vi "esp_kártya_olvasó.vi"() -> ()   [LabVIEW 2015]
uses:
  <vilib>/httpClient/POSTBuffer.vi
  <vilib>/httpClient/LabVIEWHTTPClient.lvlib
panel:
  in  "Tab Control":T1(tab)
  out "value":T2(array[cluster])
  in  "Felhasználó létrehozása":bool
  in  "Felhasználó mentése":T3
  in  "Felhasználó módosítása":bool
  in  "Felhasználó hozzáadása":T3
  out "value 2":cluster{"RFID-code":string, "time":string}[](array[cluster])
  out "Array":string[](array[string])
  out "error out":errorcluster
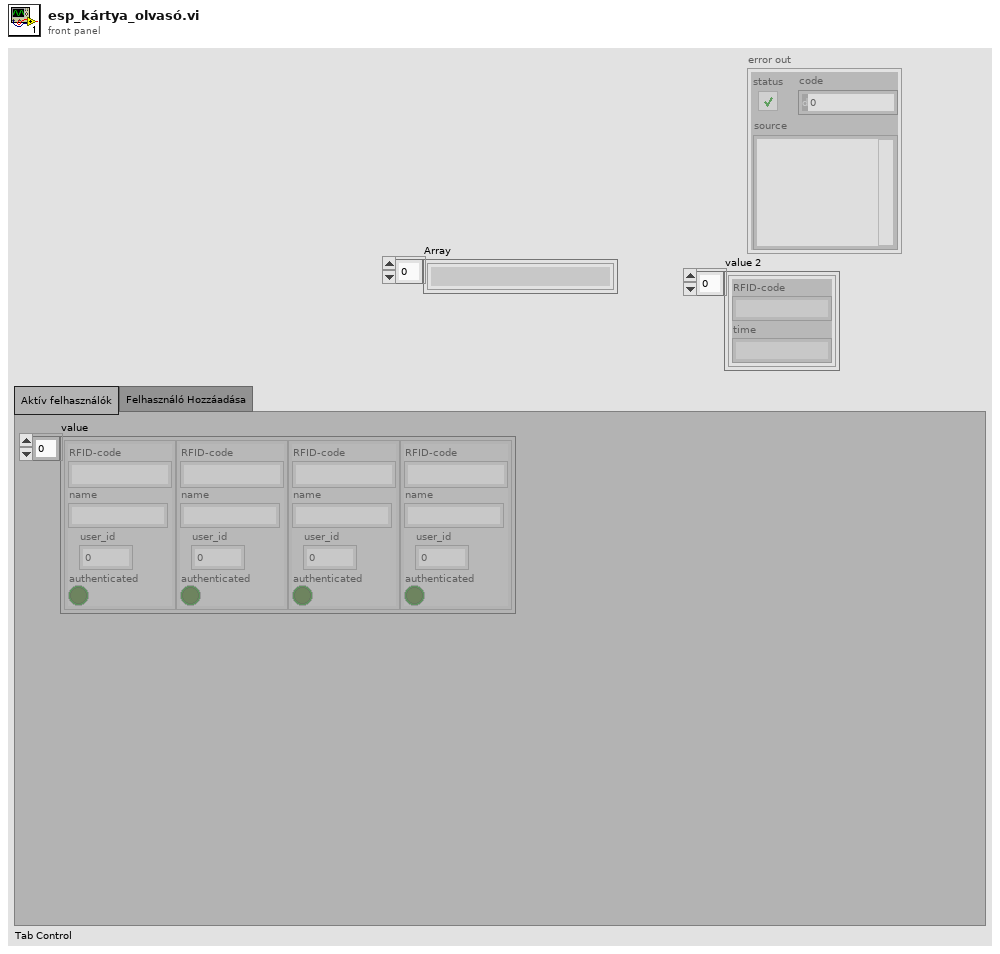
[diagram p1: front panel]
types:
  T1 = enum32{"Aktív felhasználók", "Felhasználó Hozzáadása"}
  T2 = cluster{"RFID-code":string, "name":string, "user_id":dbl, "authenticated":bool}[]
  T3 = cluster{"RFID-code":string, "name":string, "user_id":dbl, "authenticated":bool}
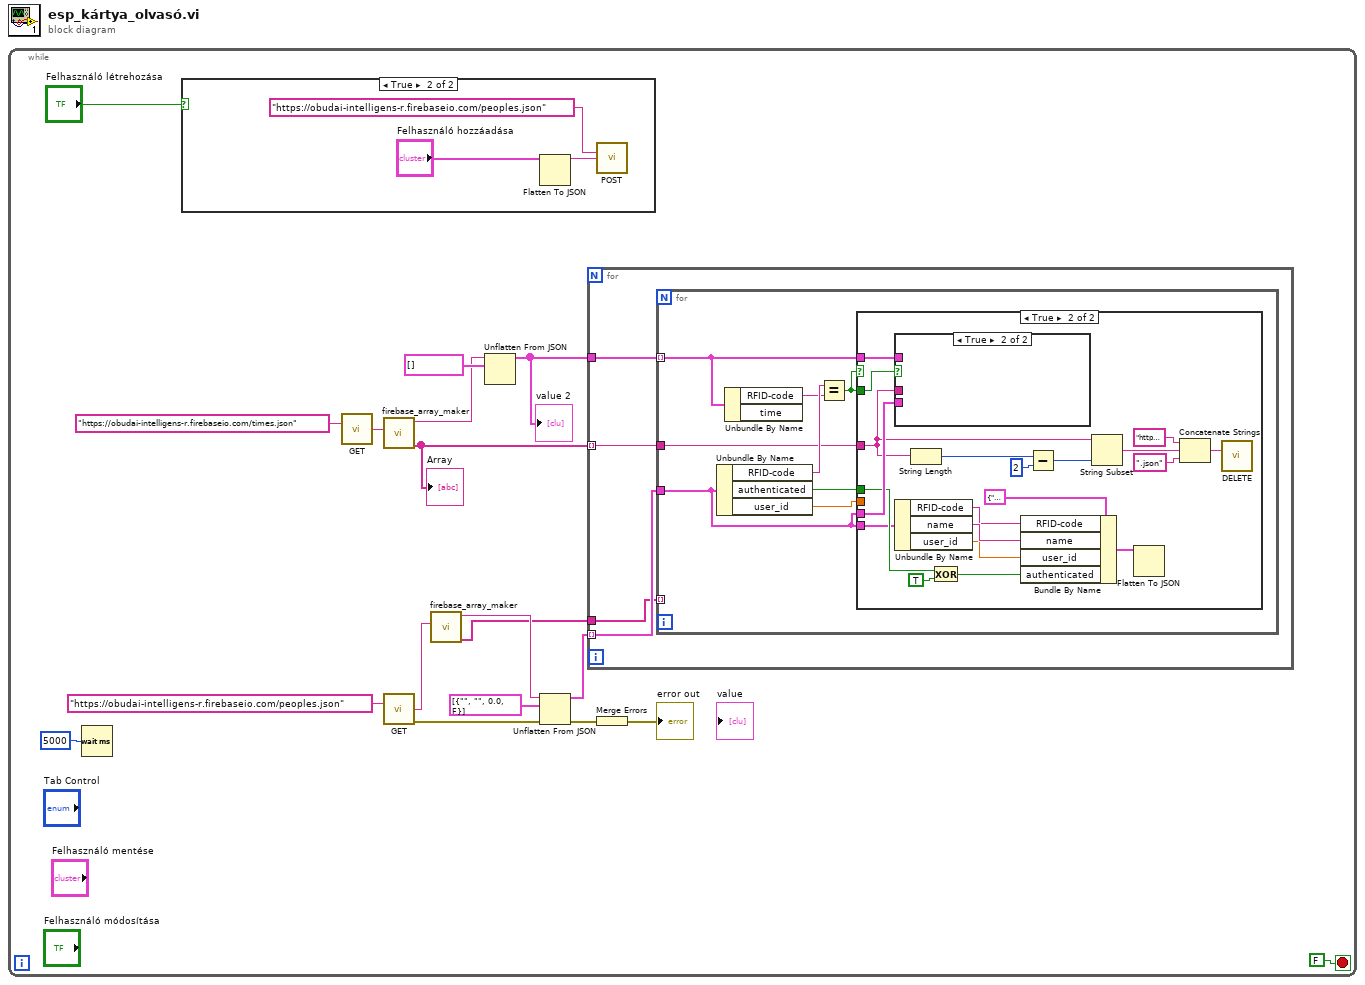
[diagram p0: block diagram]
diagram:
  n1 = while {
    stop <- FALSE stop-if-true
    n2 = Wait (ms)(milliseconds to wait=u32 5000) -> ()  [unwired: 1 out]
    n3 = case shown="True" "Felhasználó létrehozása" {
      frame False {
      }
      frame True {
        n4 = Flatten To JSON(anything="Felhasználó hozzáadása") -> (JSON string=w19:string)  [unwired: 2 in, 1 out]
        n5 = call-poly <vilib>:"POST.vi"("url"="https://obudai-intelligens-r.firebaseio.com/peoples.json", "buffer"=w19) -> ()  [unwired: 10 in, 4 out]
      }
    }
    n6 = call <vilib>:"GET.vi"("url"="https://obudai-intelligens-r.firebaseio.com/times.json") -> ("body"=w6:string)  [unwired: 11 in, 3 out]
    n7 = call "firebase_array_maker.vi"("be_string"=w6) -> ("indexek_ nevei"=w4:string[], "json ki"=w5:string)  [unwired: 9 in]
    "Array" <- w4
    n8 = call <vilib>:"GET.vi"("url"="https://obudai-intelligens-r.firebaseio.com/peoples.json") -> ("body"=w2:string, "error out"=w17:errorcluster)  [unwired: 11 in, 2 out]
    n9 = call "firebase_array_maker.vi"("be_string"=w2) -> ("indexek_ nevei"=w1:string[], "json ki"=w3:string)  [unwired: 9 in]
    n10 = Unflatten From JSON(JSON string=w5, type and defaults=cluster{"RFID-code":string, "time":string}[] [] ("Array")) -> (value=w11:cluster{"RFID-code":string, "time":string}[])  [unwired: 5 in, 1 out]
    "value 2" <- w11
    n11 = Unflatten From JSON(JSON string=w3, type and defaults=T2 [{"RFID-code"="", "name"="", "user_id"=0.0, "authenticated"=FALSE}] ("Array"), error in (no error)=w17) -> (value=w10:T2, error out=w14:errorcluster)  [unwired: 4 in]
    n12 = for {
      tunnel: w11 -> [w25]
      tunnel: w10 -> [w24] mode=indexing
      tunnel: w4 -> [w23] mode=indexing
      tunnel: w1 -> [w22]
      n13 = for {
        tunnel: w25 -> [w30] mode=indexing
        tunnel: w24 -> [w26]
        tunnel: w23 -> [w29]
        tunnel: w22 -> [_] mode=indexing
        n14 = Unbundle By Name(w26) -> ("RFID-code"=w33:string, "authenticated"=w31:bool, "user_id"=w27:dbl)
        n15 = Unbundle By Name(w30) -> ("RFID-code"=w32:string)  [unwired: 1 out]
        n16 = Equal?(x=w33, y=w32) -> (x = y?=w28:bool)
        n17 = case shown="True" w28 {
          tunnel: w31 -> [_ w42]
          tunnel: w26 -> [_ w53]
          tunnel: w30 -> [_ w52]
          tunnel: w29 -> [_ w44]
          tunnel: w28 -> [_ w51]
          tunnel: w27 -> [_ _]
          tunnel: w26 -> [_ w38]
          frame False {
          }
          frame True {
            n18 = case shown="True" w51 {
              tunnel: w53 -> [_ _]
              tunnel: w52 -> [_ _]
              tunnel: w44 -> [_ _]
              frame False {
              }
              frame True {
              }
            }
            n19 = Unbundle By Name(w38) -> ("RFID-code"=w35:string, "name"=w37:string, "user_id"=w36:dbl)
            n20 = String Length(string=w44) -> (length=w49:i32)
            n21 = Exclusive Or(1:TRUE ("y"), 2:w42) -> (0:w39:bool)
            n22 = Bundle By Name(cluster=T3 {"RFID-code"="", "name"="", "user_id"=0.0, "authenticated"=FALSE}, "RFID-code"=w35, "name"=w37, "user_id"=w36, "authenticated"=w39) -> (w34:T3)
            n23 = Subtract(x=w49, y=2) -> (x-y=w47:i32)
            n24 = String Subset(string=w44, length (rest)=w47) -> (substring=w45:string)  [unwired: 1 in]
            n25 = Flatten To JSON(anything=w34) -> ()  [unwired: 2 in, 2 out]
            n26 = Concatenate Strings("https://obudai-intelligens-r.firebaseio.com/times/" ("url"), w45, ".json" ("string")) -> (w43:string)
            n27 = call <vilib>:"DELETE.vi"("url"=w43) -> ()  [unwired: 11 in, 4 out]
          }
        }
      }
    }
    n28 = Merge Errors(w14) -> (→"error out":errorcluster)
  }
